vi "shift_instruction.vi"(10 "Instruction In":T1, 11 "Offset":i32) -> (3 "Instruction Out":T1)   [LabVIEW 2013]
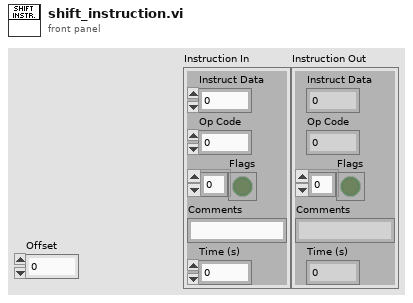
[diagram p1: front panel]
types:
  T1 = cluster{"Instruct Data":i32, "Op Code":i32, "Flags":bool[], "Comments":string, "Time (s)":dbl}
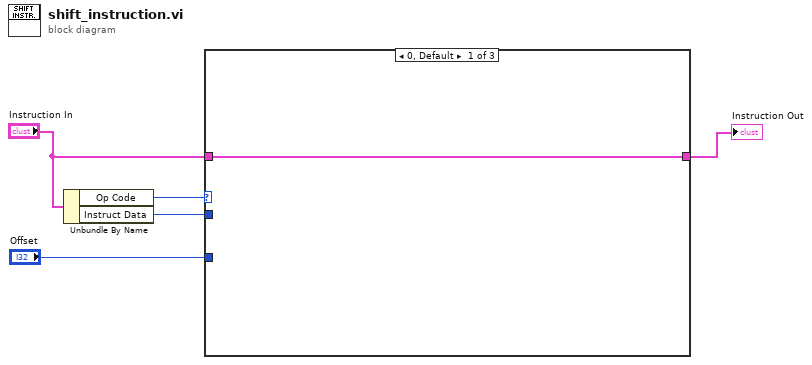
[diagram p0: block diagram]
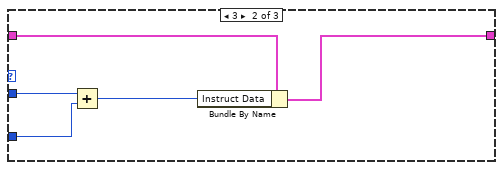
[diagram p2: hidden frame]
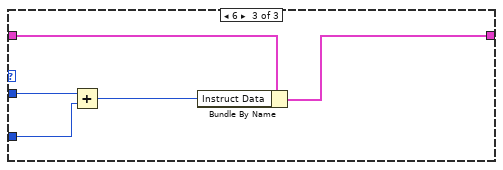
[diagram p3: hidden frame]
diagram:
  n1 = Unbundle By Name("Instruction In") -> ("Op Code"=w5:i32, "Instruct Data"=w3:i32)
  n2 = case shown="0, Default" w5 {
    tunnel: "Instruction In" -> [w6 w11 w16]
    tunnel: w3 -> [_ w9 w14]
    tunnel: "Offset" -> [_ w10 w15]
    tunnel: [w6 w7 w12] -> w1
    frame 0, Default {
    }
    frame 3 {
      n3 = Add(x=w9, y=w10) -> (x+y=w8:i32)
      n4 = Bundle By Name(cluster=w11, "Instruct Data"=w8) -> (w7:T1)
    }
    frame 6 {
      n5 = Add(x=w14, y=w15) -> (x+y=w13:i32)
      n6 = Bundle By Name(cluster=w16, "Instruct Data"=w13) -> (w12:T1)
    }
  }
  "Instruction Out" <- w1
